vi "launcherScreen.vi"(8 "Error In":errorcluster) -> (0 "Error Out":errorcluster, 1 "isSimulation?":bool, 2 "Application Path Cluster":T1, 3 "Software Name":string)   [LabVIEW 2018]
uses:
  controls/pathCluster.ctl
  b4469f8c-ff8e-4e5f-8a7c-ea0af0ade6e0.vi
panel:
  out "Status":string
  out "Software Name :":string
  out "Company Name :":string
  # "@ 2026 Thomas Technologies. All rights reserved"
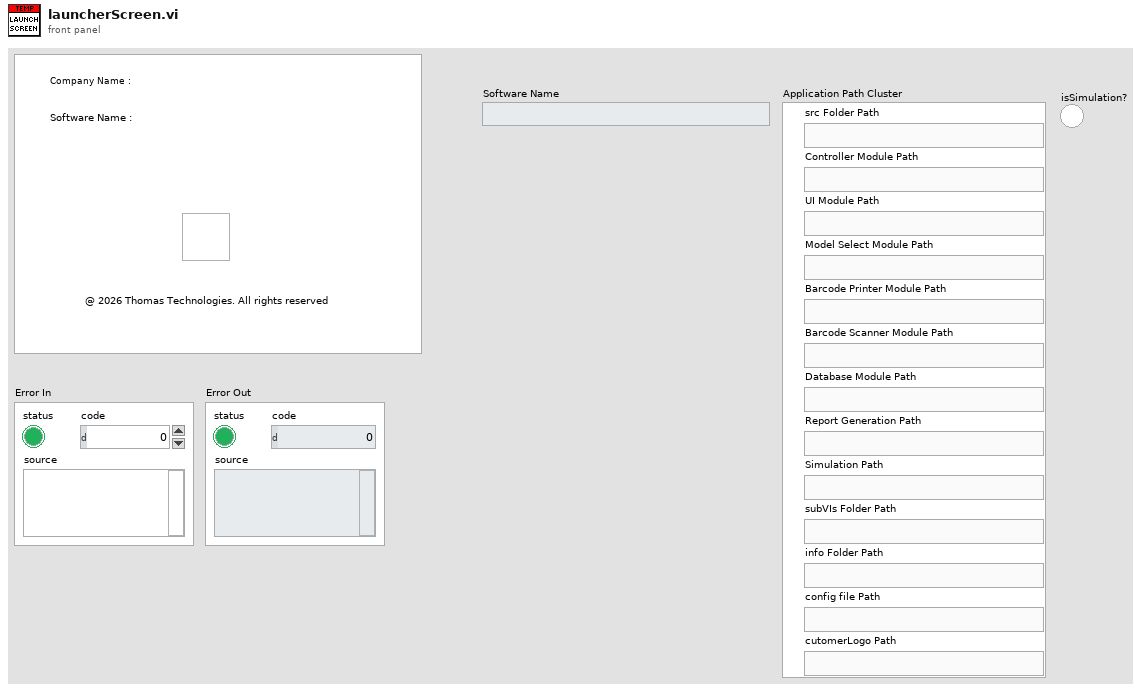
[diagram p1: front panel]
types:
  T1 = typedef "pathCluster.ctl" = cluster{"src Folder Path":path, "Controller Module Path":path, "UI Module Path":path, "Model Select Module Path":path, "Barcode Printer Module Path":path, "Barcode Scanner Module Path":path, "Database Module Path":path, "Report Generation Path":path, "Simulation Path":path, "subVIs Folder Path":path, "info Folder Path":path, "config file Path":path, "cutomerLogo Path":path}
  T2 = enum32{"Invalid", "Standard", "Closed", "Hidden", "Minimized", "Maximized"}
  T3 = enum32{"invalid app kind", "Development System", "Run Time System", "Student Edition", "Embedded LabVIEW", "Evaluation", "Custom"}
  T4 = cluster{"Core":cluster{"Current VI Reference":refnum<vi>, "Close Panel on Exit?":bool}, "Company Name":string, "Software Name":string, "Status":string, "isSimulation?":bool, "Application Path Cluster":T1}
  T5 = cluster{"Current VI Reference":refnum<vi>, "Close Panel on Exit?":bool}
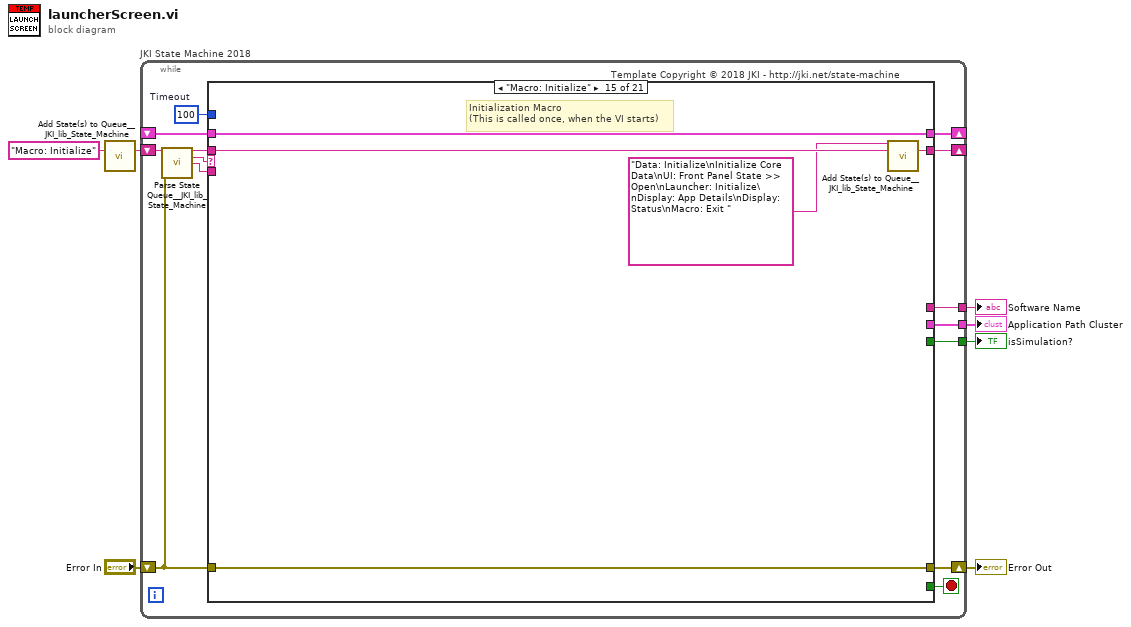
[diagram p0: block diagram]
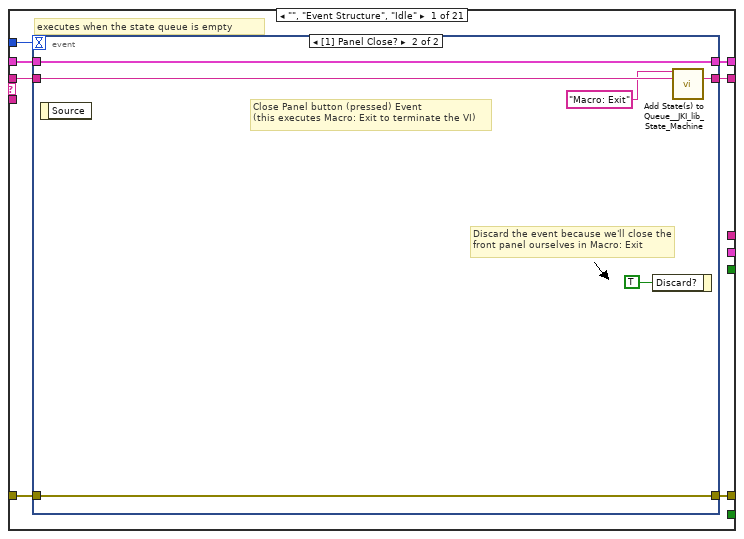
[diagram p2: hidden frame]
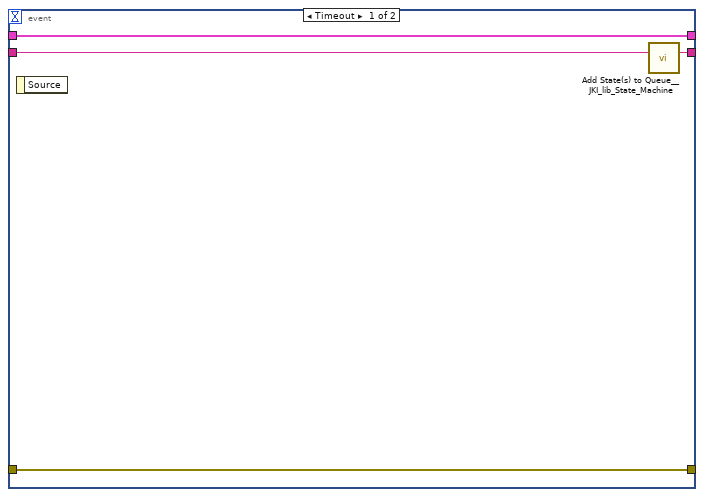
[diagram p3: hidden frame]
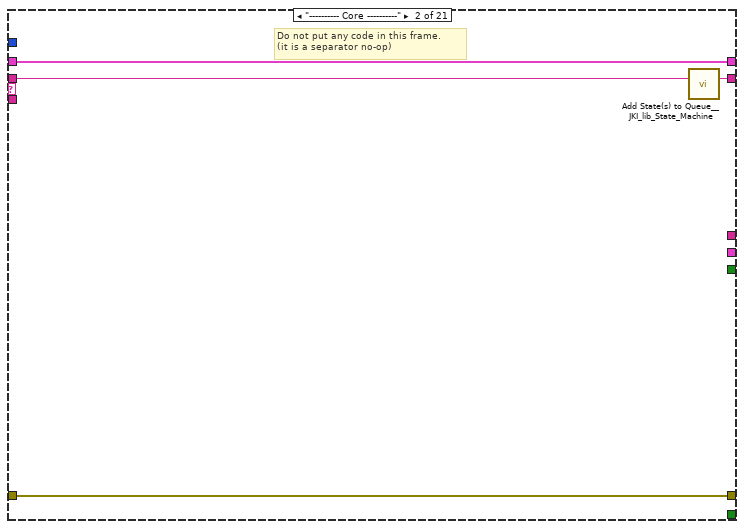
[diagram p4: hidden frame]
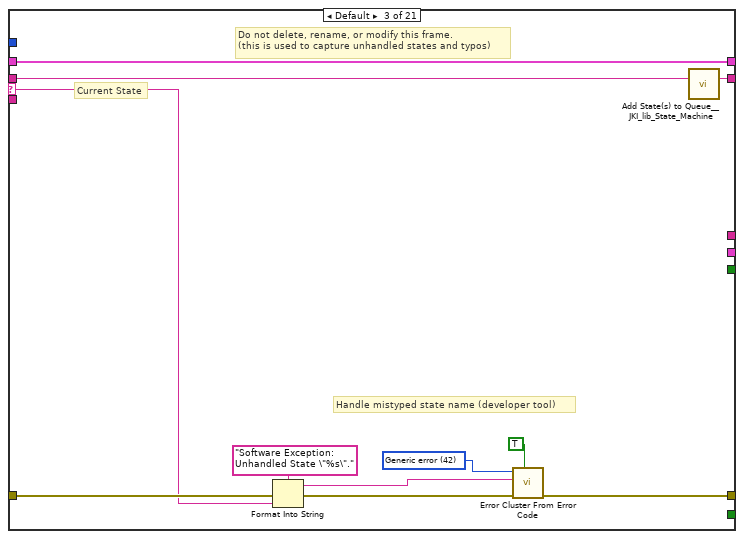
[diagram p5: hidden frame]
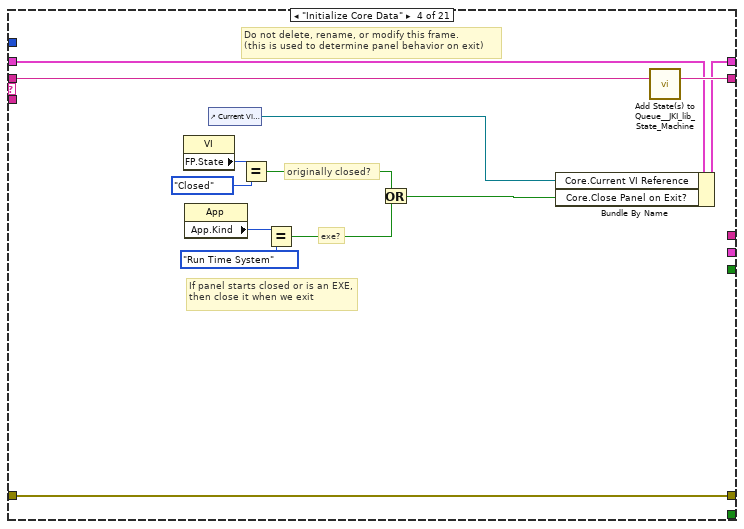
[diagram p6: hidden frame]
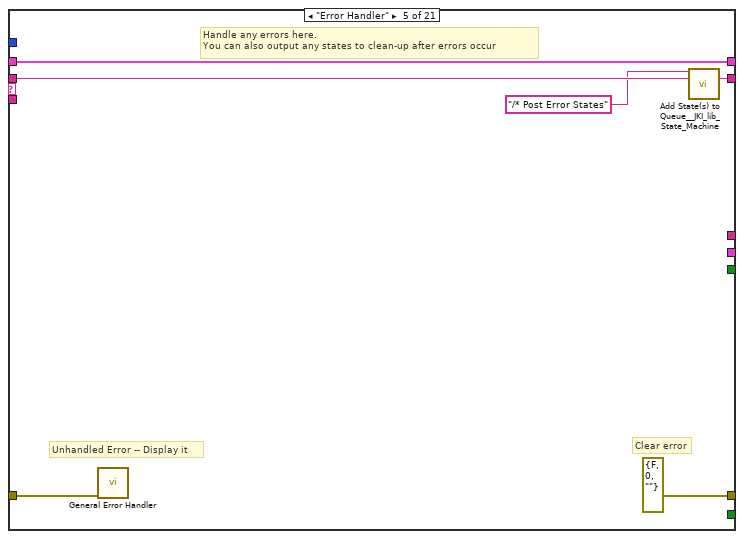
[diagram p7: hidden frame]
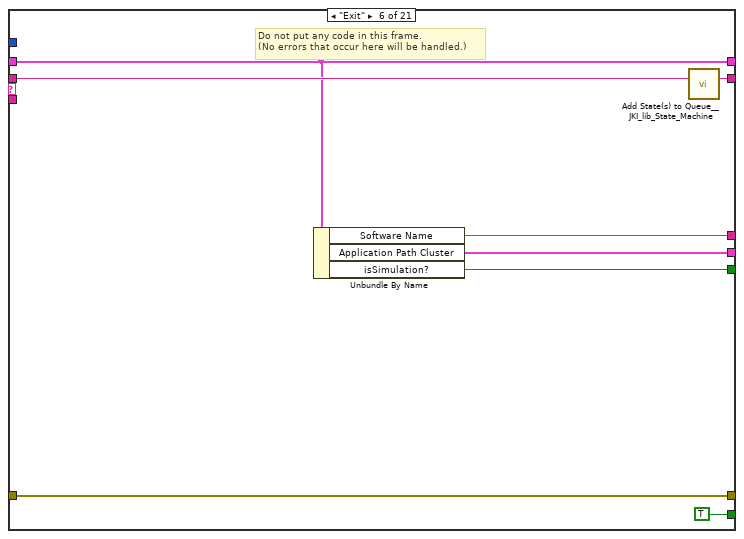
[diagram p8: hidden frame]
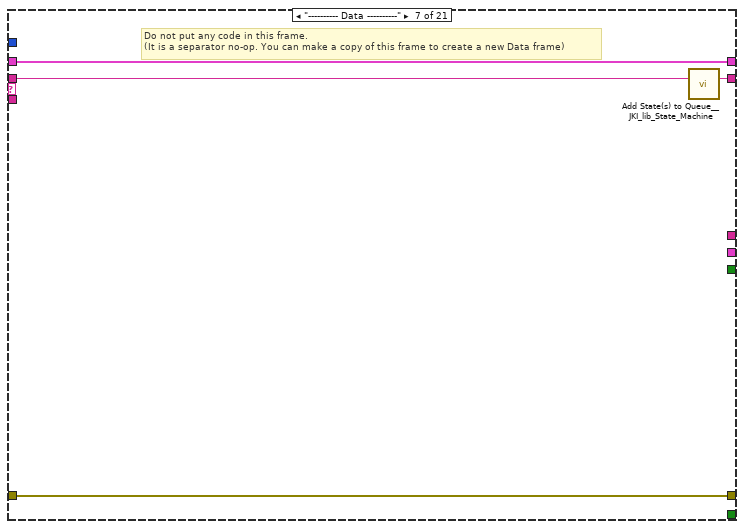
[diagram p9: hidden frame]
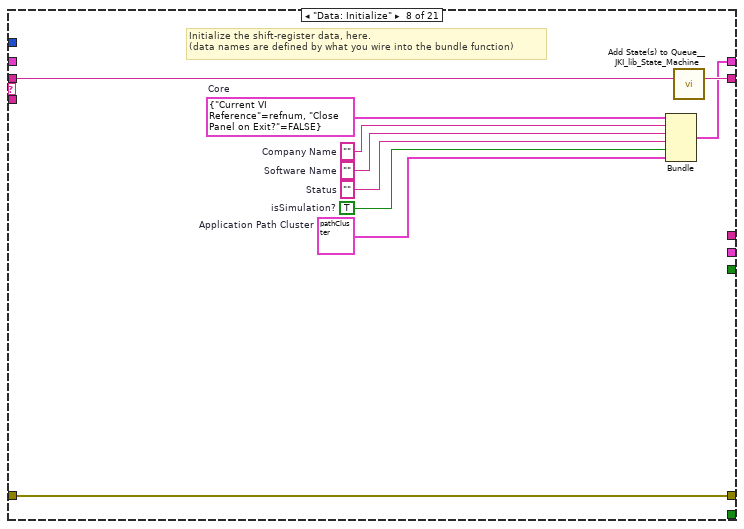
[diagram p10: hidden frame]
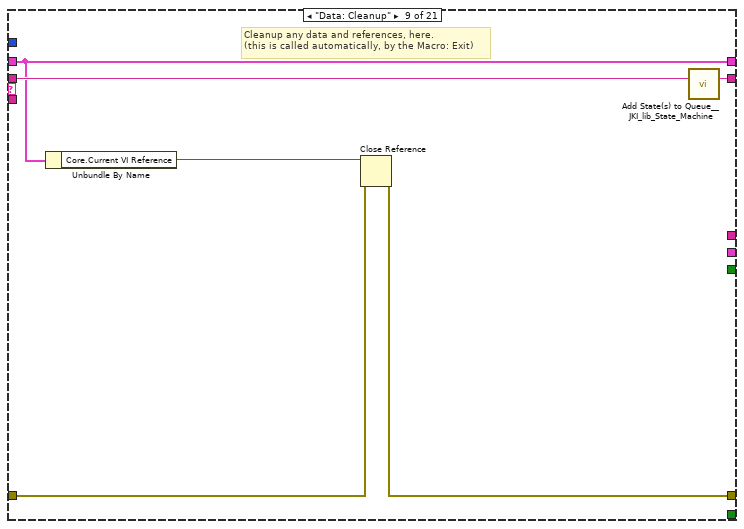
[diagram p11: hidden frame]
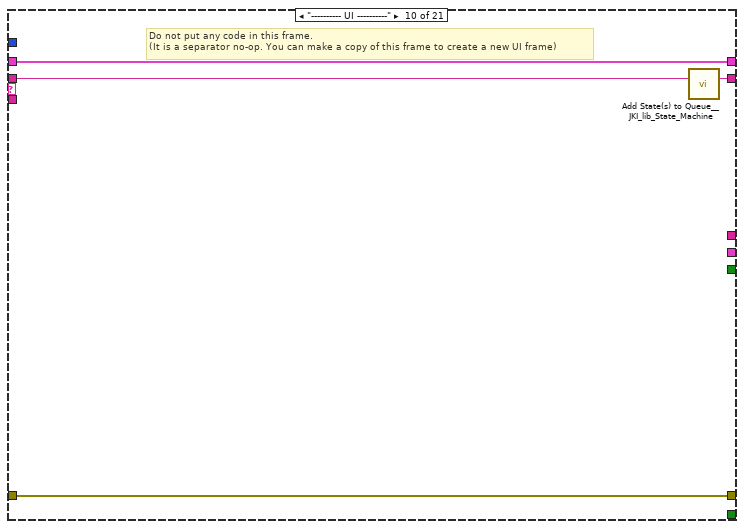
[diagram p12: hidden frame]
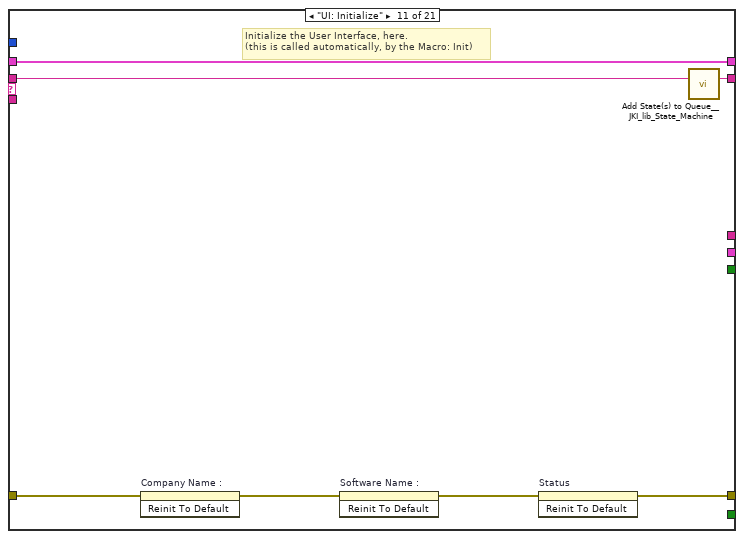
[diagram p13: hidden frame]
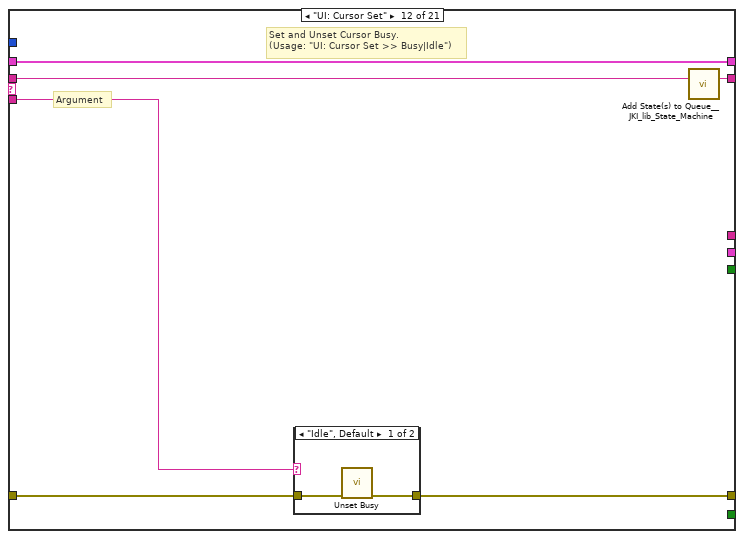
[diagram p14: hidden frame]
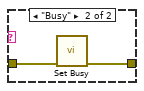
[diagram p15: hidden frame]
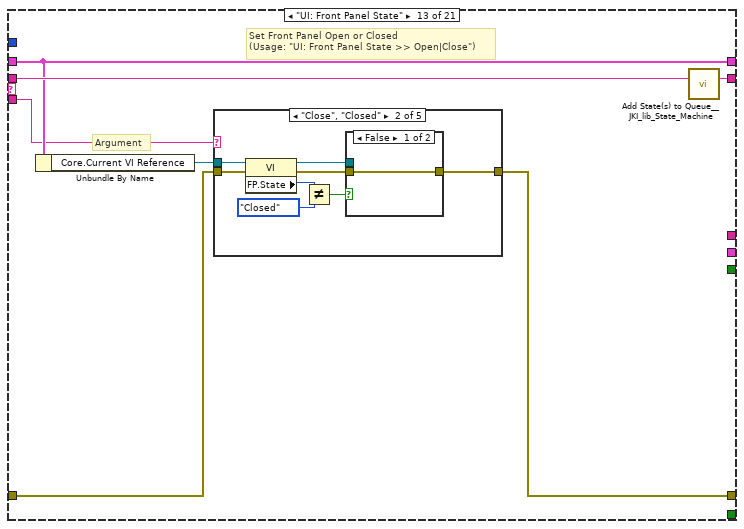
[diagram p16: hidden frame]
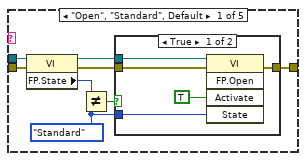
[diagram p17: hidden frame]
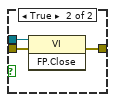
[diagram p19: hidden frame]
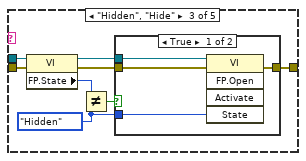
[diagram p20: hidden frame]
diagram:
  n1 = call <vilib>:"Add State(s) to Queue__JKI_lib_State_Machine.vi"("State(s) in (\"\")"="Macro: Initialize") -> ("States Out"=w7:string)  [unwired: 14 in]
  n2 = while "JKI State Machine 2018" {
    shift-right: [w14] -> _
    shift-left: _ -> [w13]
    shift-right: [w17] -> w4
    shift-left: "Error In" -> [w11]
    shift-right: [w16] -> _
    shift-left: w7 -> [w18]
    tunnel: [w10] -> w3
    tunnel: [w9] -> w2
    tunnel: [w8] -> w1
    stop <- w15 stop-if-true
    w12 = 100  # Timeout
    # "Template Copyright © 2018 JKI - http://jki.net/state-machine"
    n3 = call <vilib>:"Parse State Queue__JKI_lib_State_Machine.vi"("State Queue"=w18, "Error In (no error)"=w11) -> ("Remaining States"=w20:string, "Current State"=w21:string, "Arguments"=w19:string)  [unwired: 11 in]
    n4 = case shown="\"Macro: Initialize\"" w21 {
      selector: w21 -> [_ _ w43 _ _ _ _ _ _ _ _ _ _ _ _ _ _ _ _ _ _]
      tunnel: w20 -> [w28 w42 w47 w66 w72 w80 w84 w94 w100 w104 w111 w117 w128 w197 w202 w212 w216 w229 w233 w239 w246]
      tunnel: w19 -> [_ _ _ _ _ _ _ _ _ _ _ w112 w122 _ _ _ _ _ _ _ _]
      tunnel: w13 -> [w26 w39 w45 w59 w69 w76 w81 _ w95 w101 w109 w115 w124 w194 w199 w209 w213 w227 w230 w236 w244]
      tunnel: [w25 w40 w49 w63 errorcluster {"status"=FALSE, "code"=0, "source"=""} ("error out") w78 w82 w91 w96 w102 w105 w113 w125 w195 w200 w210 w214 w222 w231 w237 w241] -> w17
      tunnel: w11 -> [w24 w40 w48 w63 w68 w78 w82 w91 w97 w102 w108 w114 w126 w195 w200 w210 w214 w217 w231 w237 w242]
      tunnel: [w27 w41 w46 w65 w71 w79 w83 w93 w99 w103 w110 w116 w127 w196 w201 w211 w215 w228 w232 w238 w245] -> w16
      tunnel: [_ _ _ _ _ TRUE _ _ _ _ _ _ _ _ _ _ _ _ _ _ _] -> w15
      tunnel: [w23 w39 w45 w64 w69 w76 w81 w92 w95 w101 w109 w115 w124 w194 w199 w209 w213 w226 w230 w236 w244] -> w14
      tunnel: w12 -> [w22 _ _ _ _ _ _ _ _ _ _ _ _ _ _ _ _ _ _ _ _]
      tunnel: [_ _ _ _ _ w75 _ _ _ _ _ _ _ _ _ _ _ _ _ _ _] -> w10
      tunnel: [_ _ _ _ _ w74 _ _ _ _ _ _ _ _ _ _ _ _ _ _ _] -> w9
      tunnel: [_ _ _ _ _ w73 _ _ _ _ _ _ _ _ _ _ _ _ _ _ _] -> w8
      frame "", "Event Structure", "Idle" {
        # "executes when the state queue is empty"
        n5 = event shown="[1] Panel Close?" {
          selector: _ -> [_ _]
          dyn-events: _ -> [_ _]
          timeout: w22 -> [_ _]
          tunnel: w28 -> [w32 w38]
          tunnel: [w31 w37] -> w27
          tunnel: w26 -> [w29 w35]
          tunnel: [w30 w36] -> w25
          tunnel: w24 -> [w30 w36]
          tunnel: [w29 w35] -> w23
          event Timeout {
            n6 = event-data() -> ()  [unwired: 1 in, 1 out]
            n7 = call <vilib>:"Add State(s) to Queue__JKI_lib_State_Machine.vi"("State(s) in (\"\")"=w32) -> ("States Out"=w31:string)  [unwired: 14 in]
          }
          event Panel Close? {
            # "Discard the event because we'll close the front panel ourselves in Macro: Exit"
            # "Close Panel button (pressed) Event\n(this executes Macro: Exit to terminate the VI)"
            n8 = event-data() -> ()  [unwired: 1 in, 1 out]
            n9 = event-data("Discard?"=TRUE) -> ()  [unwired: 1 in, 1 out]
            n10 = call <vilib>:"Add State(s) to Queue__JKI_lib_State_Machine.vi"("State(s) in Front (\"\")"="Macro: Exit", "State(s) in (\"\")"=w38) -> ("States Out"=w37:string)  [unwired: 13 in]
          }
        }
      }
      frame "---------- Core ----------" {
        # "Do not put any code in this frame.\n(it is a separator no-op)"
        n11 = call <vilib>:"Add State(s) to Queue__JKI_lib_State_Machine.vi"("State(s) in (\"\")"=w42) -> ("States Out"=w41:string)  [unwired: 14 in]
      }
      frame Default {
        w52 = 42 items=["No error", "Argument error", "Memory is full", "Out of zone", "End of file", "File already open", "Generic file I/O error", "File not found", "File permission error", "Disk is full", "Duplicate path", "Too many files open", "System feature not enabled", "Resource file not found", "Cannot add resource", "Resource not found", "Image not found", "Image memory error", "Pen does not exist", "Config type invalid", "Config token not found", "Config parse error", "Config memory error", "Bad external code format", "Bad external code offset", "External code not present", "Null window", "Destroy window error", "Null menu", "Print aborted", "Bad print record", "Print driver error", "Windows error during printing", "Memory error during printing", "Print dialog error", "Generic print error", "Invalid device refnum", "Device not found", "Device parameter error", "Device unit error", "Cannot open device", "Device call aborted", "Generic error", "Cancelled by user", "Object ID too low", "Object ID too high", "Object not in heap", "Unknown heap", "Unknown object (invalid DefProc)", "Unknown object (DefProc not in table)", "Message out of range", "Invalid (null) method", "Unknown message", "Manager call not supported", "Bad address", "Network operation in progress", "Network operation timed out", "Connection is busy", "Network attribute not supported", "Network error", "Address in use", "System out of memory", "Connection aborted", "Connection refused", "Not connected", "Already connected", "Connection closed", "Initialization error (interapplication manager)", "Bad occurrence", "Wait on unbound occurrence handler", "Occurrence queue overflow", "Datalog type conflict", "Unused", "Unrecognized type (interapplication manager)", "Memory corrupt", "Failed to make temporary DLL", "Old CIN version", "Drag socket not found", "Failed to load drop-object", "Failed to register OLE object", "Failed to release OLE object", "Format specifier type mismatch", "Unknown format specifier", "Too few format specifiers", "Too many format specifiers", "Scan failed", "Newer CIN version", "Error converting to variant", "Runtime menu error", "Password tampered", "Variant attribute not found", "Incompatible variant data type", "Event data is not available", "Event Store is not present", "Occurrence is not found", "Event Queue is not created", "Event info is not available", "Refnum passed is NULL", "Error retrieving Class GUID", "Error retrieving CoClass GUID", "Error retrieving TypeLib GUID.", "Bad built application magic bytes.", "Specific driver is different from the specific driver associated with the Logical Name.", "There is no session opened to the class driver.", "Max Error", "MAX - Error with config objects", "MAX - Error loading configuration", "MAX - Group not supported"]
        # "Current State"
        # "Do not delete, rename, or modify this frame.\n(this is used to capture unhandled states and typos)"
        # "Handle mistyped state name (developer tool)"
        n12 = Format Into String(format string="Software Exception: Unhandled State \"%s\"." ("message"), error in=w48, w43) -> (resulting string=w51:string, error out=w50:errorcluster)  [unwired: 1 in]
        n13 = call <vilib>:"Error Cluster From Error Code.vi"("show call chain? (False)"=TRUE, "error in (no error)"=w50, "error message (\"\")"=w51, "error code (0)"=w52) -> ("error out"=w49:errorcluster)  [unwired: 5 in]
        n14 = call <vilib>:"Add State(s) to Queue__JKI_lib_State_Machine.vi"("State(s) in (\"\")"=w47) -> ("States Out"=w46:string)  [unwired: 14 in]
      }
      frame "Initialize Core Data" {
        # "Do not delete, rename, or modify this frame.\n(this is used to determine panel behavior on exit)"
        # "originally closed?"
        # "exe?"
        # "If panel starts closed or is an EXE, then close it when we exit"
        n15 = property class="VI"() -> ("FP.State"=w56:T2)  [unwired: 2 in, 2 out]
        n16 = property class="App"() -> ("App.Kind"=w62:T3)  [unwired: 2 in, 2 out]
        n17 = control-ref of="Current VI Reference"() -> (w57:refnum<vi>)
        n18 = Equal?(x=w56, y=T2."Closed" ("Front Panel Window:State")) -> (x = y?=w54:bool)
        n19 = Equal?(x=w62, y=T3."Run Time System" ("Application:Kind")) -> (x = y?=w60:bool)
        n20 = Or(x=w54, y=w60) -> (x .or. y?=w58:bool)
        n21 = Bundle By Name(cluster=w59, "Core.Current VI Reference"=w57, "Core.Close Panel on Exit?"=w58) -> (w64:T4)
        n22 = call <vilib>:"Add State(s) to Queue__JKI_lib_State_Machine.vi"("State(s) in (\"\")"=w66) -> ("States Out"=w65:string)  [unwired: 14 in]
      }
      frame "Error Handler" {
        # "Unhandled Error -- Display it"
        # "Handle any errors here.\nYou can also output any states to clean-up after errors occur"
        # "Clear error"
        n23 = call <vilib>:"General Error Handler.vi"("error in (no error)"=w68) -> ()  [unwired: 10 in, 5 out]
        n24 = call <vilib>:"Add State(s) to Queue__JKI_lib_State_Machine.vi"("State(s) in Front (\"\")"="/* Post Error States", "State(s) in (\"\")"=w72) -> ("States Out"=w71:string)  [unwired: 13 in]
      }
      frame "Exit" {
        # "Do not put any code in this frame.\n(No errors that occur here will be handled.)"
        n25 = Unbundle By Name(w76) -> ("Software Name"=w75:string, "Application Path Cluster"=w74:T1, "isSimulation?"=w73:bool)
        n26 = call <vilib>:"Add State(s) to Queue__JKI_lib_State_Machine.vi"("State(s) in (\"\")"=w80) -> ("States Out"=w79:string)  [unwired: 14 in]
      }
      frame "---------- Data ----------" {
        # "Do not put any code in this frame.\n(It is a separator no-op. You can make a copy of this frame to create a new Data frame)"
        n27 = call <vilib>:"Add State(s) to Queue__JKI_lib_State_Machine.vi"("State(s) in (\"\")"=w84) -> ("States Out"=w83:string)  [unwired: 14 in]
      }
      frame "Data: Initialize" {
        w85 = TRUE  # isSimulation?
        w86 = T1 {"src Folder Path"=path "", "Controller Module Path"=path "", "UI Module Path"=path "", "Model Select Module Path"=path "", "Barcode Printer Module Path"=path "", "Barcode Scanner Module Path"=path "", "Database Module Path"=path "", "Report Generation Path"=path "", "Simulation Path"=path "", "subVIs Folder Path"=path "", "info Folder Path"=path "", "config file Path"=path "", "cutomerLogo Path"=path ""}  # Application Path Cluster
        w88 = ""  # Software Name
        w87 = ""  # Status
        w89 = ""  # Company Name
        w90 = T5 {"Current VI Reference"=refnum, "Close Panel on Exit?"=FALSE}  # Core
        # "Initialize the shift-register data, here.\n(data names are defined by what you wire into the bundle function)"
        n28 = Bundle("Core"=w90, "Company Name"=w89, "Software Name"=w88, "Status"=w87, "isSimulation?"=w85, "Application Path Cluster"=w86) -> (w92:T4)  [unwired: 1 in]
        n29 = call <vilib>:"Add State(s) to Queue__JKI_lib_State_Machine.vi"("State(s) in (\"\")"=w94) -> ("States Out"=w93:string)  [unwired: 14 in]
      }
      frame "Data: Cleanup" {
        # "Cleanup any data and references, here.\n(this is called automatically, by the Macro: Exit)"
        n30 = Unbundle By Name(w95) -> ("Core.Current VI Reference"=w98:refnum<vi>)
        n31 = Close Reference(reference=w98, error in (no error)=w97) -> (error out=w96:errorcluster)
        n32 = call <vilib>:"Add State(s) to Queue__JKI_lib_State_Machine.vi"("State(s) in (\"\")"=w100) -> ("States Out"=w99:string)  [unwired: 14 in]
      }
      frame "---------- UI ----------" {
        # "Do not put any code in this frame.\n(It is a separator no-op. You can make a copy of this frame to create a new UI frame)"
        n33 = call <vilib>:"Add State(s) to Queue__JKI_lib_State_Machine.vi"("State(s) in (\"\")"=w104) -> ("States Out"=w103:string)  [unwired: 14 in]
      }
      frame "UI: Initialize" {
        # "Initialize the User Interface, here.\n(this is called automatically, by the Macro: Init)"
        n34 = invoke on="Company Name :" class="Str" method="Reinit To Default"(error in=w108) -> (error out=w107:errorcluster)  [unwired: 2 in, 2 out]
        n35 = invoke on="Software Name :" class="Str" method="Reinit To Default"(error in=w107) -> (error out=w106:errorcluster)  [unwired: 2 in, 2 out]
        n36 = invoke on="Status" class="Str" method="Reinit To Default"(error in=w106) -> (error out=w105:errorcluster)  [unwired: 2 in, 2 out]
        n37 = call <vilib>:"Add State(s) to Queue__JKI_lib_State_Machine.vi"("State(s) in (\"\")"=w111) -> ("States Out"=w110:string)  [unwired: 14 in]
      }
      frame "UI: Cursor Set" {
        # "Argument"
        # "Set and Unset Cursor Busy.\n(Usage: \"UI: Cursor Set >> Busy|Idle\")"
        n38 = case shown="\"Idle\", Default" w112 {
          tunnel: w114 -> [w119 w121]
          tunnel: [w118 w120] -> w113
          frame "Idle", Default {
            n39 = call <vilib>:"Unset Busy.vi"("error in (no error)"=w119) -> ("error out"=w118:errorcluster)  [unwired: 10 in]
          }
          frame "Busy" {
            n40 = call <vilib>:"Set Busy.vi"("error in (no error)"=w121) -> ("error out"=w120:errorcluster)  [unwired: 9 in, 1 out]
          }
        }
        n41 = call <vilib>:"Add State(s) to Queue__JKI_lib_State_Machine.vi"("State(s) in (\"\")"=w117) -> ("States Out"=w116:string)  [unwired: 14 in]
      }
      frame "UI: Front Panel State" {
        # "Argument"
        # "Set Front Panel Open or Closed\n(Usage: \"UI: Front Panel State >> Open|Close\")"
        n42 = Unbundle By Name(w124) -> ("Core.Current VI Reference"=w123:refnum<vi>)
        n43 = case shown="\"Close\", \"Closed\"" w122 {
          tunnel: w126 -> [w134 w149 w160 w173 w186]
          tunnel: [w136 w150 w162 w175 w188] -> w125
          tunnel: w123 -> [w135 w147 w161 w174 w187]
          frame "Open", "Standard", Default {
            w129 = T2."Standard" ("State")
            n44 = property class="VI"(reference=w135, error in=w134) -> (reference out=w132:refnum<vi>, error out=w133:errorcluster, "FP.State"=w131:T2)
            n45 = Not Equal?(x=w131, y=w129) -> (x != y?=w130:bool)
            n46 = case shown="True" w130 {
              tunnel: [w140 w142] -> w136
              tunnel: w133 -> [w139 w142]
              tunnel: w132 -> [w138 _]
              tunnel: w129 -> [w137 _]
              frame True {
                n47 = invoke class="VI" method="FP.Open"(reference=w138, error in=w139, "Activate"=TRUE, "State"=w137) -> (error out=w140:errorcluster)  [unwired: 1 in, 4 out]
              }
              frame False {
              }
            }
          }
          frame "Close", "Closed" {
            n48 = property class="VI"(reference=w147, error in=w149) -> (reference out=w146:refnum<vi>, error out=w148:errorcluster, "FP.State"=w144:T2)
            n49 = Not Equal?(x=w144, y=T2."Closed" ("Front Panel Window:State")) -> (x != y?=w143:bool)
            n50 = case shown="False" w143 {
              tunnel: [w151 w154] -> w150
              tunnel: w148 -> [w151 w153]
              tunnel: w146 -> [_ w152]
              frame False {
              }
              frame True {
                n51 = invoke class="VI" method="FP.Close"(reference=w152, error in=w153) -> (error out=w154:errorcluster)  [unwired: 1 in, 2 out]
              }
            }
          }
          frame "Hidden", "Hide" {
            w155 = T2."Hidden" ("State")
            n52 = property class="VI"(reference=w161, error in=w160) -> (reference out=w158:refnum<vi>, error out=w159:errorcluster, "FP.State"=w157:T2)
            n53 = Not Equal?(x=w157, y=w155) -> (x != y?=w156:bool)
            n54 = case shown="True" w156 {
              tunnel: [w166 w167] -> w162
              tunnel: w159 -> [w165 w167]
              tunnel: w158 -> [w164 _]
              tunnel: w155 -> [w163 _]
              frame True {
                n55 = invoke class="VI" method="FP.Open"(reference=w164, error in=w165, "State"=w163) -> (error out=w166:errorcluster)  [unwired: 2 in, 4 out]
              }
              frame False {
              }
            }
          }
          frame "Minimize", "Minimized" {
            w168 = T2."Minimized" ("State")
            n56 = property class="VI"(reference=w174, error in=w173) -> (reference out=w171:refnum<vi>, error out=w172:errorcluster, "FP.State"=w170:T2)
            n57 = Not Equal?(x=w170, y=w168) -> (x != y?=w169:bool)
            n58 = case shown="True" w169 {
              tunnel: [w179 w180] -> w175
              tunnel: w172 -> [w178 w180]
              tunnel: w171 -> [w177 _]
              tunnel: w168 -> [w176 _]
              frame True {
                n59 = invoke class="VI" method="FP.Open"(reference=w177, error in=w178, "State"=w176) -> (error out=w179:errorcluster)  [unwired: 2 in, 4 out]
              }
              frame False {
              }
            }
          }
          frame "Maximize", "Maximized" {
            w181 = T2."Maximized" ("State")
            n60 = property class="VI"(reference=w187, error in=w186) -> (reference out=w184:refnum<vi>, error out=w185:errorcluster, "FP.State"=w183:T2)
            n61 = Not Equal?(x=w183, y=w181) -> (x != y?=w182:bool)
            n62 = case shown="True" w182 {
              tunnel: [w192 w193] -> w188
              tunnel: w185 -> [w191 w193]
              tunnel: w184 -> [w190 _]
              tunnel: w181 -> [w189 _]
              frame True {
                n63 = invoke class="VI" method="FP.Open"(reference=w190, error in=w191, "State"=w189) -> (error out=w192:errorcluster)  [unwired: 2 in, 4 out]
              }
              frame False {
              }
            }
          }
        }
        n64 = call <vilib>:"Add State(s) to Queue__JKI_lib_State_Machine.vi"("State(s) in (\"\")"=w128) -> ("States Out"=w127:string)  [unwired: 14 in]
      }
      frame "---------- Macro ----------" {
        # "Do not put any code in this frame.\n(It is a separator no-op. You can make a copy of this frame to create a new Macro frame)"
        n65 = call <vilib>:"Add State(s) to Queue__JKI_lib_State_Machine.vi"("State(s) in (\"\")"=w197) -> ("States Out"=w196:string)  [unwired: 14 in]
      }
      frame "Macro: Initialize" {
        # "Initialization Macro\n(This is called once, when the VI starts)"
        n66 = call <vilib>:"Add State(s) to Queue__JKI_lib_State_Machine.vi"("State(s) in Front (\"\")"="Data: Initialize\nInitialize Core Data\nUI: Front Panel State >> Open\nLauncher: Initialize\nDisplay: App Details\nDisplay: Status\nMacro: Exit ", "State(s) in (\"\")"=w202) -> ("States Out"=w201:string)  [unwired: 13 in]
      }
      frame "Macro: Exit" {
        # "Exit Macro\n(This is called once, when the VI exits)"
        n67 = Unbundle By Name(w209) -> ("Core.Close Panel on Exit?"=w208:bool)
        n68 = Select(t="UI: Front Panel State >> Close", s=w208, f="") -> (s? t:f=w205:string)
        n69 = call <vilib>:"Add State(s) to Queue__JKI_lib_State_Machine.vi"("State(s) in (\"\")"=w205, "State(s) at Back (\"\")"="Data: Cleanup\nExit") -> ("States Out"=w203:string)  [unwired: 13 in]
        n70 = call <vilib>:"Add State(s) to Queue__JKI_lib_State_Machine.vi"("State(s) in Front (\"\")"=w203, "State(s) in (\"\")"=w212) -> ("States Out"=w211:string)  [unwired: 13 in]
      }
      frame "---------- Launcher ----------" {
        # "Template Separator\n(You can make a copy of, or modify, this frame)"
        n71 = call <vilib>:"Add State(s) to Queue__JKI_lib_State_Machine.vi"("State(s) in (\"\")"=w216) -> ("States Out"=w215:string)  [unwired: 14 in]
      }
      frame "Launcher: Initialize" {
        # "Template Separator\n(You can make a copy of, or modify, this frame)"
        n72 = call "getPaths.vi"("Error In"=w217) -> ("Error Out"=w223:errorcluster, "Application Path Cluster"=w224:T1)  [unwired: 9 in]
        n73 = Unbundle By Name(w224) -> ("config file Path"=w221:path)
        n74 = call "readAppConfigFile.vi"("Error In"=w223, "App Config File Path"=w221) -> ("Error Out"=w222:errorcluster, "isSimulation?"=w218:bool, "Software Name"=w219:string, "Company Name"=w220:string)  [unwired: 6 in]
        n75 = Bundle By Name(cluster=w227, "Status"="Loading... Please Wait...", "Application Path Cluster"=w224, "Company Name"=w220, "Software Name"=w219, "isSimulation?"=w218) -> (w226:T4)
        n76 = call <vilib>:"Add State(s) to Queue__JKI_lib_State_Machine.vi"("State(s) in (\"\")"=w229) -> ("States Out"=w228:string)  [unwired: 14 in]
      }
      frame "---------- Display ----------" {
        # "Template Separator\n(You can make a copy of, or modify, this frame)"
        n77 = call <vilib>:"Add State(s) to Queue__JKI_lib_State_Machine.vi"("State(s) in (\"\")"=w233) -> ("States Out"=w232:string)  [unwired: 14 in]
      }
      frame "Display: App Details" {
        # "Template Separator\n(You can make a copy of, or modify, this frame)"
        n78 = Unbundle By Name(w236) -> ("Company Name"=→"Company Name :":string, "Software Name"=→"Software Name :":string)
        n79 = call <vilib>:"Add State(s) to Queue__JKI_lib_State_Machine.vi"("State(s) in (\"\")"=w239) -> ("States Out"=w238:string)  [unwired: 14 in]
      }
      frame "Display: Status" {
        # "Template Separator\n(You can make a copy of, or modify, this frame)"
        n80 = Unbundle By Name(w244) -> ("Status"=→"Status":string)
        n81 = call "Stall Data Flow.vim"("value in"=w242, "milliseconds to wait"=u32 1000) -> ("value out"=w241:errorcluster)  [unwired: 1 out]
        n82 = call <vilib>:"Add State(s) to Queue__JKI_lib_State_Machine.vi"("State(s) in (\"\")"=w246) -> ("States Out"=w245:string)  [unwired: 14 in]
      }
    }
  }
  "Error Out" <- w4
  "Application Path Cluster" <- w2
  "Software Name" <- w3
  "isSimulation?" <- w1
